vi "TrajectoryCreateAbsoluteSwerveReef.vi"(4 "Spline Type":T9, 5 "MaxVelocity Fraction":dbl=0.8 format="%17.3f", 6 "Max Cent Accel INCHES/SEC^2":dbl=40.0 format="%20.1f", 7 "MaxAcceleration INCHES/SEC^2":dbl=60.0 format="%17.1f", 8 "End Pose  ENG":T1={"TRANSLATION"={"X"=0.0, "Y"=0.0}, "ROTATION"={"VALUE"=0.0, "COS"=1.0, "SIN"=0.0}} {"ROTATION"."SIN" format="%13.4f"; "ROTATION"."COS" format="%13.4f"; "ROTATION"."VALUE" format="%13.4f"; "TRANSLATION"."Y" format="%14.3f"; "TRANSLATION"."X" format="%14.3f"}, 9 "Current Pose SI":T1={"TRANSLATION"={"X"=0.0, "Y"=0.0}, "ROTATION"={"VALUE"=0.0, "COS"=1.0, "SIN"=0.0}} {"ROTATION"."SIN" format="%13.4f"; "ROTATION"."COS" format="%13.4f"; "ROTATION"."VALUE" format="%13.4f"; "TRANSLATION"."Y" format="%14.3f"; "TRANSLATION"."X" format="%14.3f"}, 10 "Max Velocity Ft/Sec":dbl=13.0 format="%17.3f", 11 "SWERVE_DRIVE_KINEMATICS":T4 {"SavedModuleStates"."Angle"."SIN" format="%13.4f"; "SavedModuleStates"."Angle"."COS" format="%13.4f"; "SavedModuleStates"."Angle"."VALUE" format="%13.4f"; "PrevCoR"."Y" format="%14.3f"; "PrevCoR"."X" format="%14.3f"; "Modules"."Y" format="%14.3f"; "Modules"."X" format="%14.3f"}) -> (0 "Trajectory  creation error":errorcluster, 1 "Absolute Trajectory":T7 {"States"."POSE"."ROTATION"."SIN" format="%13.4f"; "States"."POSE"."ROTATION"."COS" format="%13.4f"; "States"."POSE"."ROTATION"."VALUE" format="%13.4f"; "States"."POSE"."TRANSLATION"."Y" format="%14.3f"; "States"."POSE"."TRANSLATION"."X" format="%14.3f"; "TotalTImeSecs" format="%20.3f"}, 3 "TotalTImeSecs":dbl)   [LabVIEW 2023]
doc: "Create absolute trajectory for swerve drive robot. Outputs trajectry both to an indicator and a global variable."
uses:
  <vilib>/Rock Robotics/WPI/ThirdParty/JAS_Junk/TrajLib/Enum/TRAJECTORY_SPLINE_TYPE_ENUM.ctl
  <vilib>/Rock Robotics/WPI/ThirdParty/JAS_Junk/TrajLib/TypeDef/TRAJECTORY.ctl
  <vilib>/Rock Robotics/WPI/ThirdParty/JAS_Junk/TrajLib/TypeDef/TRAJ_STATE.ctl
  <vilib>/Rock Robotics/WPI/ThirdParty/JAS_Junk/TrajLib/TypeDef/POSE2D.ctl
  <vilib>/Rock Robotics/WPI/ThirdParty/JAS_Junk/TrajLib/TypeDef/TRANSLATION2D.ctl
  <vilib>/Rock Robotics/WPI/ThirdParty/JAS_Junk/TrajLib/TypeDef/ROTATION2D.ctl
  <vilib>/Rock Robotics/WPI/ThirdParty/JAS_Junk/TrajLib/TypeDef/SWERVE_DRIVE_KINEMATICS.ctl
  <vilib>/Analysis/Matrix/Datatypes/RealMatrix.ctl
  <vilib>/Rock Robotics/WPI/ThirdParty/JAS_Junk/TrajLib/TypeDef/SWERVE_DRIVE_MODULE_STATE.ctl
  <vilib>/Rock Robotics/WPI/ThirdParty/JAS_Junk/TrajLib/Util_CalcDist.vi
  <vilib>/Rock Robotics/WPI/ThirdParty/JAS_Junk/TrajLib/Rotation2d_CreateXY.vi
  <vilib>/Rock Robotics/WPI/ThirdParty/JAS_Junk/TrajLib/Rotation2d_CreateAngle.vi
  <vilib>/Rock Robotics/WPI/ThirdParty/JAS_Junk/TrajLib/MathUtil_InputModulus.vi
  <vilib>/Rock Robotics/WPI/ThirdParty/JAS_Junk/TrajLib/SwerveDriveKinematicsConstraint_New.vi
  <vilib>/Rock Robotics/WPI/ThirdParty/JAS_Junk/TrajLib/TrajectoryConfig_AddConstraint.vi
  <vilib>/Rock Robotics/WPI/ThirdParty/JAS_Junk/TrajLib/CentripetalAccelConstraint_New.vi
  TrajectoryGlobals.vi
  <vilib>/Rock Robotics/WPI/ThirdParty/JAS_Junk/TrajLib/Trajectory_Library.lvlib
  <vilib>/Analysis/Matrix/NI_Matrix.lvlib
panel:
  in  "Use Swerve Drive\nKinematic\nConstraint":bool=TRUE
  in  "Use Centripetal\nAcceleration\nConstaint":bool=TRUE
  # "TRAJECTORY CONFIGURATION"
  # "TRAJECTORY DEFINITION"
  # "Feet, Rad"
  # "Meters, Rad"
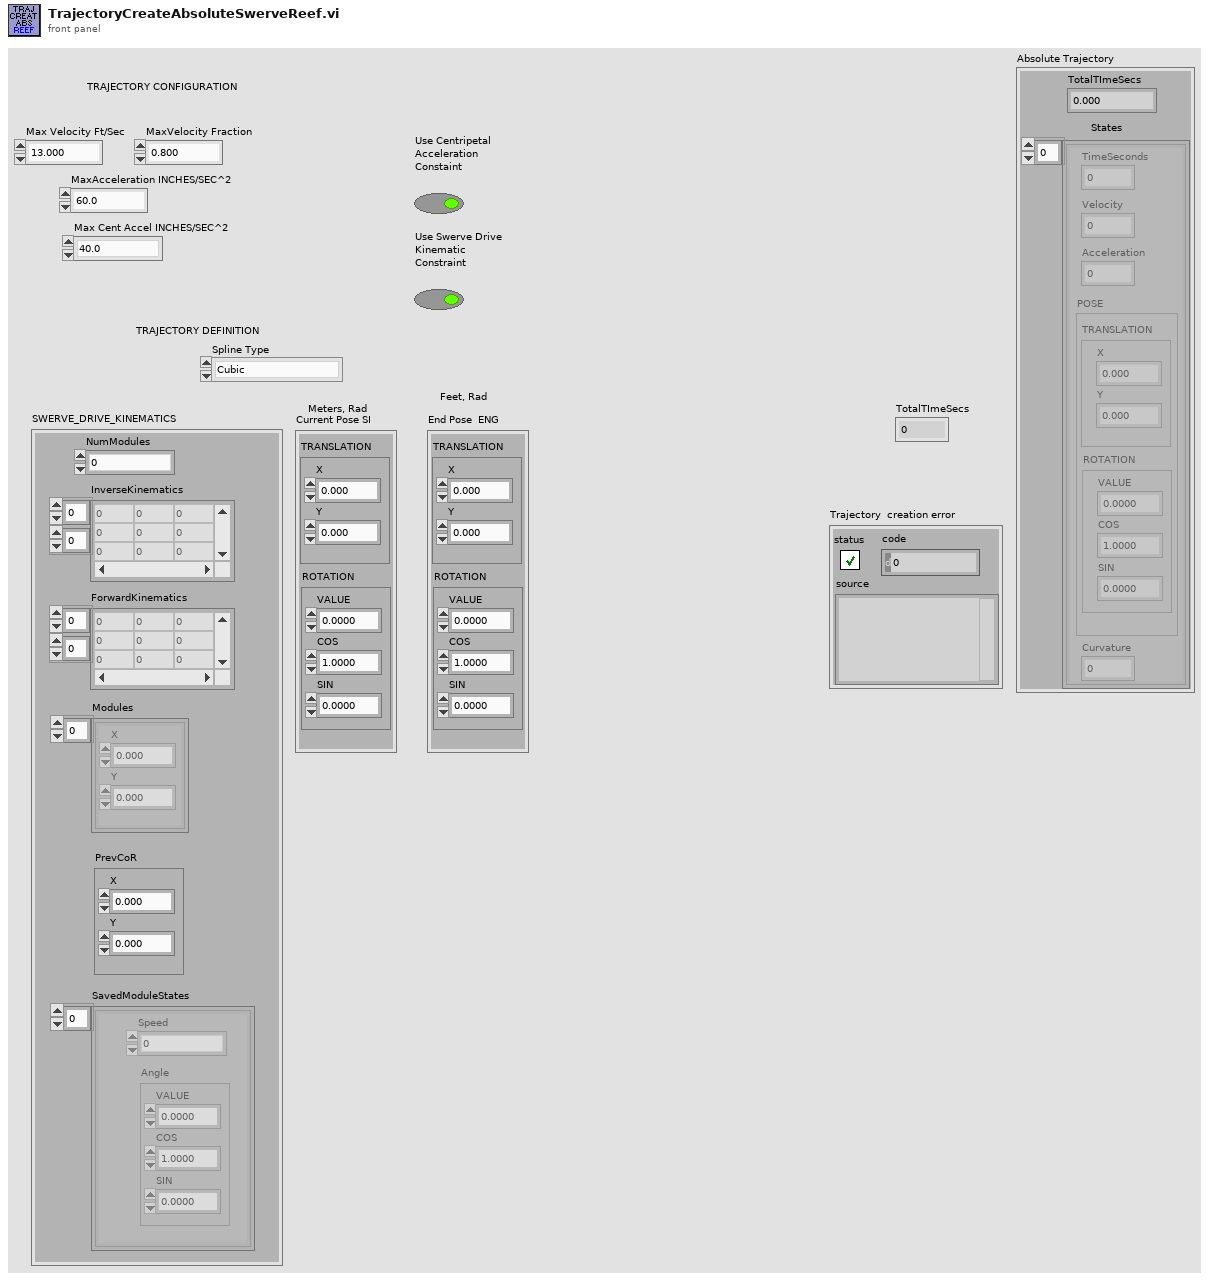
[diagram p1: front panel]
types:
  T1 = typedef "Trajectory_Library.lvlib/POSE2D.ctl" = cluster{"TRANSLATION":T2, "ROTATION":T3}
  T2 = typedef "Trajectory_Library.lvlib/TRANSLATION2D.ctl" = cluster{"X":dbl, "Y":dbl}
  T3 = typedef "Trajectory_Library.lvlib/ROTATION2D.ctl" = cluster{"VALUE":dbl, "COS":dbl, "SIN":dbl}
  T4 = typedef "Trajectory_Library.lvlib/SWERVE_DRIVE_KINEMATICS.ctl" = cluster{"NumModules":i32, "InverseKinematics":T5, "ForwardKinematics":T5, "Modules":T2[], "PrevCoR":T2, "SavedModuleStates":T6[]}
  T5 = typedef "NI_Matrix.lvlib/RealMatrix.ctl" = dbl[][]
  T6 = typedef "Trajectory_Library.lvlib/SWERVE_DRIVE_MODULE_STATE.ctl" = cluster{"Speed":dbl, "Angle":T3}
  T7 = typedef "Trajectory_Library.lvlib/TRAJECTORY.ctl" = cluster{"TotalTImeSecs":dbl, "States":T8[]}
  T8 = typedef "Trajectory_Library.lvlib/TRAJ_STATE.ctl" = cluster{"TimeSeconds":dbl, "Velocity":dbl, "Acceleration":dbl, "POSE":T1, "Curvature":dbl}
  T9 = typedef "Trajectory_Library.lvlib/TRAJECTORY_SPLINE_TYPE_ENUM.ctl" = enum16{"Cubic", "Cubic With Weights", "Quintic", "Quintic With Weights"}
  T10 = typedef "Trajectory_Library.lvlib/WEIGHTED_WAYPOINT.ctl" = cluster{"TRANSLATION":T2, "ROTATION":T3, "SCALAR":dbl}
  T11 = typedef "Trajectory_Library.lvlib/TRAJ_CONFIG.ctl" = cluster{"MaxVelocity":dbl, "Max Acceleration":dbl, "StartVelocity":dbl, "End Velocity":dbl, "Reversed":bool, "Constraints":variant[]}
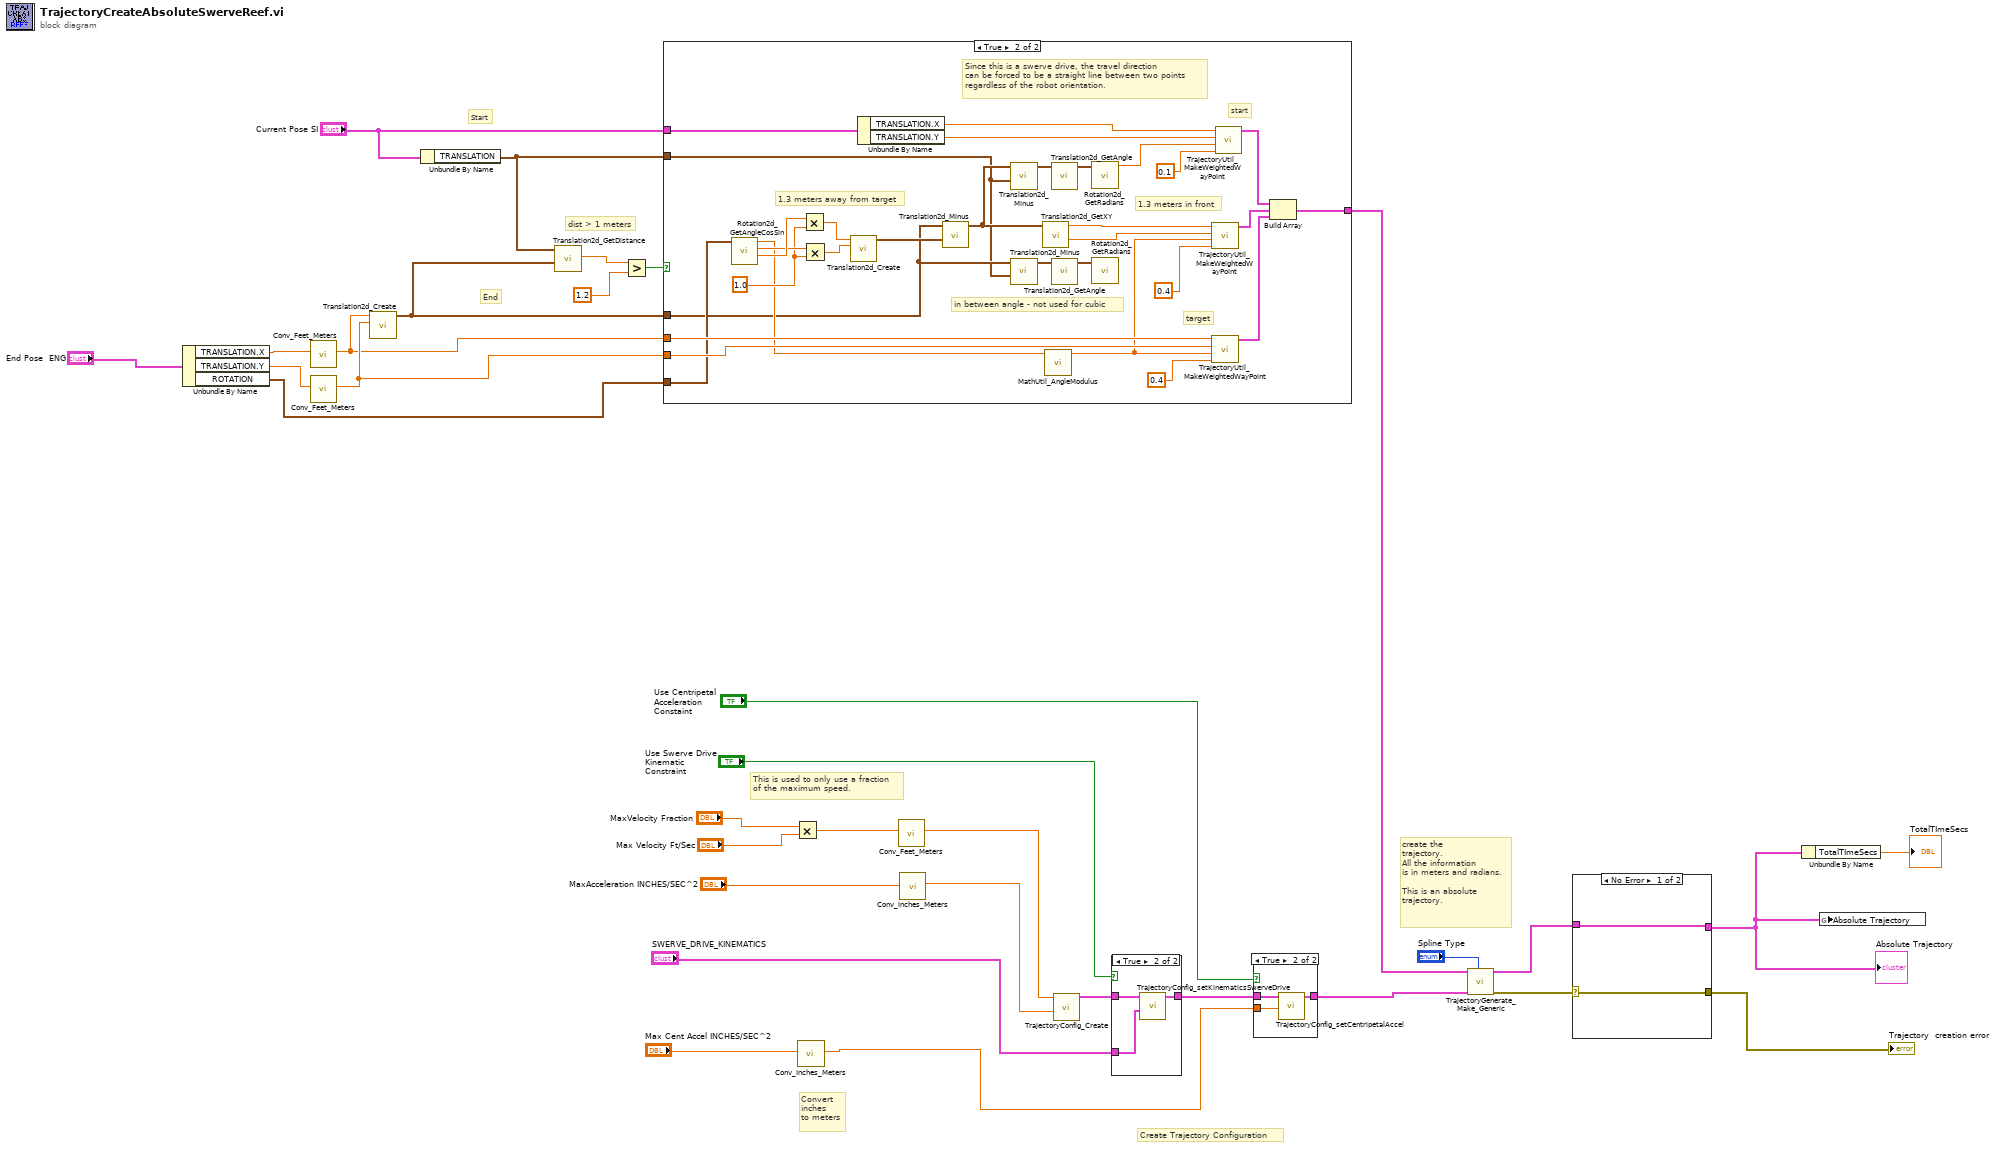
[diagram p0: block diagram]
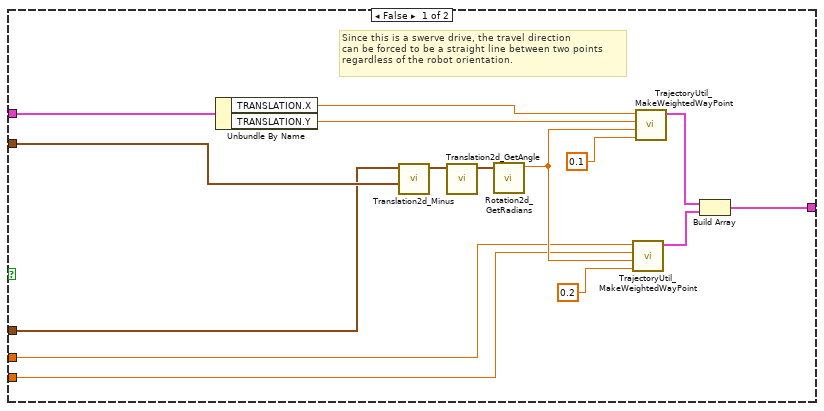
[diagram p2: hidden frame]
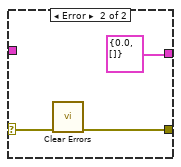
[diagram p3: hidden frame]
diagram:
  # "End"
  # "Start"
  # "dist > 1 meters"
  # "This is used to only use a fraction\nof the maximum speed."
  # "Convert\ninches\nto meters"
  # "create the\ntrajectory.\nAll the information\nis in meters and radians.\n\nThis is an absolute \ntrajectory."
  # "Create Trajectory Configuration"
  n1 = Unbundle By Name("End Pose  ENG") -> ("TRANSLATION.X"=w17:dbl, "TRANSLATION.Y"=w16:dbl, "ROTATION"=w1:T3)
  n2 = call <vilib>:"Conv_Feet_Meters.vi"("Feet"=w17) -> ("Meters"=w5:dbl)  [unwired: 10 in]
  n3 = call <vilib>:"Conv_Feet_Meters.vi"("Feet"=w16) -> ("Meters"=w6:dbl)  [unwired: 10 in]
  n4 = call <vilib>:"Translation2d_Create.vi"("Y"=w6, "X"=w5) -> ("TRANSLATION"=w7:T2)  [unwired: 9 in]
  n5 = Unbundle By Name("Current Pose SI") -> ("TRANSLATION"=w8:T2)
  n6 = call <vilib>:"Translation2d_GetDistance.vi"("other Translation"=w7, "In Translation"=w8) -> ("Distance"=w10:dbl)  [unwired: 9 in]
  n7 = Greater?(x=w10, y=1.2) -> (0:w2:bool)
  n8 = case shown="True" w2 {
    tunnel: w8 -> [w41 w50]
    tunnel: w7 -> [w40 w51]
    tunnel: w6 -> [w38 w69]
    tunnel: w5 -> [w37 w70]
    tunnel: "Current Pose SI" -> [w36 w71]
    tunnel: [w34 w65] -> w3
    tunnel: w1 -> [_ w64]
    frame False {
      # "Since this is a swerve drive, the travel direction\ncan be forced to be a straight line between two points\nregardless of the robot orientation."
      n9 = Unbundle By Name(w36) -> ("TRANSLATION.X"=w43:dbl, "TRANSLATION.Y"=w44:dbl)
      n10 = call <vilib>:"Translation2d_Minus.vi"("other Translation"=w41, "In Translation"=w40) -> ("Out Translation"=w46:T2)  [unwired: 9 in]
      n11 = call <vilib>:"Translation2d_GetAngle.vi"("In Translation"=w46) -> ("Angle_Rotation2d"=w47:T3)  [unwired: 10 in]
      n12 = call <vilib>:"Rotation2d_GetRadians.vi"("in ROTATION"=w47) -> ("AngleRadians"=w48:dbl)  [unwired: 10 in]
      n13 = call <vilib>:"TrajectoryUtil_MakeWeightedWayPoint.vi"("Weight"=0.2, "Travel Angle Radians"=w48, "Y_M"=w38, "X_M"=w37) -> ("WEIGHTED_WAYPOINT"=w45:T10)  [unwired: 7 in]
      n14 = call <vilib>:"TrajectoryUtil_MakeWeightedWayPoint.vi"("Weight"=0.1, "Travel Angle Radians"=w48, "Y_M"=w44, "X_M"=w43) -> ("WEIGHTED_WAYPOINT"=w42:T10)  [unwired: 7 in]
      n15 = Build Array(w42, w45) -> (w34:T10[])
    }
    frame True {
      w61 = 1.0
      # "in between angle - not used for cubic"
      # "target"
      # "1.3 meters in front"
      # "start"
      # "1.3 meters away from target"
      # "Since this is a swerve drive, the travel direction\ncan be forced to be a straight line between two points\nregardless of the robot orientation."
      n16 = call <vilib>:"Rotation2d_GetAngleCosSin.vi"("in ROTATION"=w64) -> ("Cosine"=w63:dbl, "Sine"=w62:dbl, "Angle"=w55:dbl)  [unwired: 8 in]
      n17 = Multiply(x=w63, y=w61) -> (x*y=w60:dbl)
      n18 = Multiply(x=w62, y=w61) -> (x*y=w59:dbl)
      n19 = call <vilib>:"Translation2d_Create.vi"("Y"=w59, "X"=w60) -> ("TRANSLATION"=w58:T2)  [unwired: 9 in]
      n20 = Unbundle By Name(w71) -> ("TRANSLATION.X"=w75:dbl, "TRANSLATION.Y"=w76:dbl)
      n21 = call <vilib>:"Translation2d_Minus.vi"("other Translation"=w58, "In Translation"=w51) -> ("Out Translation"=w54:T2)  [unwired: 9 in]
      n22 = call <vilib>:"Translation2d_Minus.vi"("other Translation"=w50, "In Translation"=w54) -> ("Out Translation"=w77:T2)  [unwired: 9 in]
      n23 = call <vilib>:"Translation2d_Minus.vi"("other Translation"=w50, "In Translation"=w51) -> ("Out Translation"=w52:T2)  [unwired: 9 in]
      n24 = call <vilib>:"Translation2d_GetXY.vi"("In Translation"=w54) -> ("Y"=w56:dbl, "X"=w57:dbl)  [unwired: 9 in]
      n25 = call <vilib>:"MathUtil_AngleModulus.vi"("InputAngle"=w55) -> ("ModulsAngle"=w49:dbl)  [unwired: 10 in]
      n26 = call <vilib>:"Translation2d_GetAngle.vi"("In Translation"=w77) -> ("Angle_Rotation2d"=w78:T3)  [unwired: 10 in]
      n27 = call <vilib>:"Translation2d_GetAngle.vi"("In Translation"=w52) -> ("Angle_Rotation2d"=w53:T3)  [unwired: 10 in]
      n28 = call <vilib>:"Rotation2d_GetRadians.vi"("in ROTATION"=w78) -> ("AngleRadians"=w79:dbl)  [unwired: 10 in]
      n29 = call <vilib>:"Rotation2d_GetRadians.vi"("in ROTATION"=w53) -> ()  [unwired: 10 in, 1 out]
      n30 = call <vilib>:"TrajectoryUtil_MakeWeightedWayPoint.vi"("Weight"=0.4, "Travel Angle Radians"=w49, "Y_M"=w56, "X_M"=w57) -> ("WEIGHTED_WAYPOINT"=w66:T10)  [unwired: 7 in]
      n31 = call <vilib>:"TrajectoryUtil_MakeWeightedWayPoint.vi"("Weight"=0.4, "Travel Angle Radians"=w49, "Y_M"=w69, "X_M"=w70) -> ("WEIGHTED_WAYPOINT"=w67:T10)  [unwired: 7 in]
      n32 = call <vilib>:"TrajectoryUtil_MakeWeightedWayPoint.vi"("Weight"=0.1, "Travel Angle Radians"=w79, "Y_M"=w76, "X_M"=w75) -> ("WEIGHTED_WAYPOINT"=w74:T10)  [unwired: 7 in]
      n33 = Build Array(w74, w66, w67) -> (w65:T10[])
    }
  }
  n34 = Multiply(x="MaxVelocity Fraction", y="Max Velocity Ft/Sec") -> (x*y=w22:dbl)
  n35 = call <vilib>:"Conv_Inches_Meters.vi"("INCH"="Max Cent Accel INCHES/SEC^2") -> ("Meters"=w27:dbl)  [unwired: 10 in]
  n36 = call <vilib>:"Conv_Feet_Meters.vi"("Feet"=w22) -> ("Meters"=w25:dbl)  [unwired: 10 in]
  n37 = call <vilib>:"Conv_Inches_Meters.vi"("INCH"="MaxAcceleration INCHES/SEC^2") -> ("Meters"=w26:dbl)  [unwired: 10 in]
  n38 = call <vilib>:"TrajectoryConfig_Create.vi"("MaxAcceleration"=w26, "MaxVelocity"=w25) -> ("TRAJECTORY_CONFIG"=w31:T11)  [unwired: 9 in]
  n39 = case shown="True" "Use Swerve Drive\nKinematic\nConstraint" {
    tunnel: w31 -> [w80 w83]
    tunnel: [w80 w82] -> w30
    tunnel: "SWERVE_DRIVE_KINEMATICS" -> [_ w81]
    frame False {
    }
    frame True {
      n40 = call <vilib>:"TrajectoryConfig_setKinematicsSwerveDrive.vi"("SWERVE_DRIVE_KINEMATICS"=w81, "inTRAJECTORY_CONFIG"=w83) -> ("outTRAJECTORY_CONFIG"=w82:T11)  [unwired: 9 in]
    }
  }
  n41 = case shown="True" "Use Centripetal\nAcceleration\nConstaint" {
    tunnel: w30 -> [w84 w87]
    tunnel: [w84 w86] -> w24
    tunnel: w27 -> [_ w85]
    frame False {
    }
    frame True {
      n42 = call <vilib>:"TrajectoryConfig_setCentripetalAccel.vi"("Max Cent Accel"=w85, "inTRAJECTORY_CONFIG"=w87) -> ("outTRAJECTORY_CONFIG"=w86:T11)  [unwired: 9 in]
    }
  }
  n43 = call <vilib>:"TrajectoryGenerate_Make_Generic.vi"("Spline Type"="Spline Type", "traj_config"=w24, "WeightedWayPoints"=w3) -> ("error out"=w15:errorcluster, "TRAJECTORY"=w14:T7)  [unwired: 7 in]
  n44 = case shown="No Error" w15 {
    selector: w15 -> [w88 w91]
    tunnel: w14 -> [w89 _]
    tunnel: [w89 T7 {"TotalTImeSecs"=0.0, "States"=[]} ("TRAJECTORY")] -> w12
    tunnel: [w88 w90] -> w13
    frame No Error {
    }
    frame Error {
      n45 = call <vilib>:"Clear Errors.vi"("error in (no error)"=w91) -> ("error out"=w90:errorcluster)  [unwired: 5 in, 1 out]
    }
  }
  "Trajectory  creation error" <- w13
  "Absolute Trajectory" <- w12
  n46 = Unbundle By Name(w12) -> ("TotalTImeSecs"=→"TotalTImeSecs":dbl)
  n47 = global write "TrajectoryGlobals.vi" "Absolute Trajectory"(w12) -> ()
